vi "Scale Charts.vi"(5 "window length":i32, 7 "sample rate":sgl format="%.2f", 8 "XY Grahp":refnum<vi>, 9 "IntesityChart":refnum<vi>, 10 "Waveform Chart":refnum<vi>) -> ()   [LabVIEW 2017]
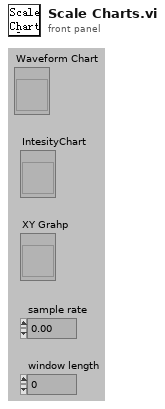
[diagram p1: front panel]
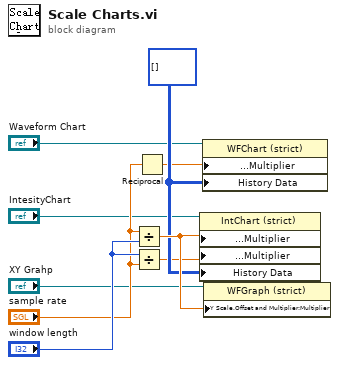
[diagram p0: block diagram]
diagram:
  w6 = i16[][] [] ("Write Attribute")
  n1 = Divide(x="sample rate", y="window length") -> (x/y=w7:sgl)
  n2 = Divide(x="window length", y="sample rate") -> (x/y=w5:sgl)
  n3 = Reciprocal(x="sample rate") -> (1/x=w4:sgl)
  n4 = property on="Property Node" class="IntChart (strict)"(reference="IntesityChart", "Y Scale.Offset and Multiplier:Multiplier"=w7, "X Scale.Offset and Multiplier:Multiplier"=w5, "History Data"=w6) -> ()  [unwired: 1 in, 2 out]
  n5 = property on="Property Node" class="WFChart (strict)"(reference="Waveform Chart", "X Scale.Offset and Multiplier:Multiplier"=w4, "History Data"=w6) -> ()  [unwired: 1 in, 2 out]
  n6 = property on="Property Node" class="WFGraph (strict)"(reference="XY Grahp", "Y Scale.Offset and Multiplier:Multiplier"=w7) -> ()  [unwired: 1 in, 2 out]
